vi "Furnace_Power.vi"(10 "Furnace Power (off)":bool) -> (2 "Status":bool)   [LabVIEW 2019]
panel:
  out "error out":errorcluster
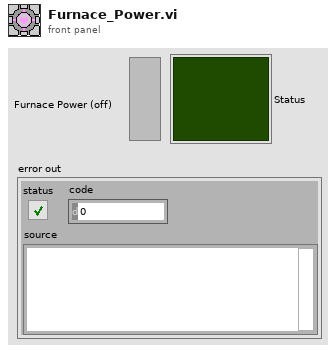
[diagram p1: front panel]
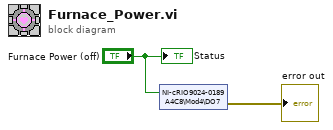
[diagram p0: block diagram]
diagram:
  n1 = shared-variable "NI-cRIO9024-0189A4C8\\Mod4\\DO7"("Furnace Power (off)") -> (error out=→"error out":errorcluster)  [unwired: 1 in]
  "Status" <- "Furnace Power (off)"
